vi "SigGen-Compute Max Level (full).vi"(0 "Waveform":T21(xcontrol), 5 "Filter":T4(xcontrol), 9 "Level":T1, 11 "error in (no error)":errorcluster, 12 "Sampling Rate (Hz)":dbl, 13 "Npts":i32) -> (10 "Level out":T1, 14 "Max Level":dbl, 15 "error out":errorcluster)   [LabVIEW 2020]
uses:
  Controls/Waveform XCtl/Waveform XCtl.xctl
  Controls/Advanced Filter XCtl/Advanced Filter XCtl.xctl
  Controls/Level XCtl/Level Data.ctl
  Controls/Level XCtl/Level Units.ctl
  Waveform VIs/Noise VIs/Noise-Globals.vi
  Controls/Level XCtl/Level XCtl.xctl
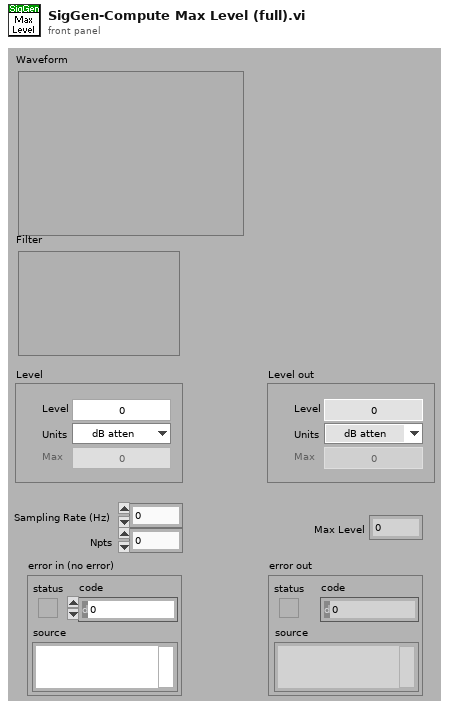
[diagram p1: front panel]
types:
  T1 = typedef "Level XCtl.xctl/Level Data.ctl" = cluster{"Level":dbl, "Units":T2, "Max":dbl, "Multiplier":dbl, "Cal File":path, "Cal":cluster{"Freq (Hz)":dbl[], "Mag (dB SPL)":dbl[], "Phase (deg)":dbl[]}}
  T2 = typedef "Level Units.ctl" = enum16{"dB atten", "dB SPL", "dB re 1 Vrms", "dB V/Hz½", "mW", "dB HL", "Volts", "dB mW"}
  T3 = typedef "Filter-Bandwidth Units.ctl" = enum16{"Linear", "Octaves", "Min-Max"}
  T4 = cluster{"Type":enum16{"Lowpass", "Highpass", "Bandpass", "Bandstop", "OFF"}, "CF (kHz)":dbl, "BW (kHz)":dbl, "Cascade":bool, "Quadrature":bool, "Scale Factor":dbl, "Stages":cluster{"IIR Filter":cluster{"filter structure":enum32{"IIR 2nd Order", "IIR 4th Order"}, "Reverse Coefficients":dbl[], "Forward Coefficients":dbl[]}, "State":dbl[]}[], "Class":enum16{"Elliptic", "Butterworth"}, "Order":i32, "BWUnits":T3}
  T5 = typedef "Waveform Enum.ctl" = enum16{"OFF", "Tone", "Noise", "Pulse Train", "File", "FM Sweep", "Chirp Train", "Complex Tone", "FM Tone", "Moving Ripple"}
  T6 = typedef "Tone Params.ctl" = cluster{"Frequency (kHz)":dbl, "Last Freq":dbl, "Last Phase":dbl}
  T7 = typedef "Pulse Train Params.ctl" = cluster{"Pulse width (us)":dbl, "Pulse rate (Hz)":dbl, "Gap (ms)":dbl, "Polarity":T8, "PT State":T9, "Asynch":bool}
  T8 = typedef "Pulse Polarity.ctl" = enum16{"POS", "NEG", "POS-NEG", "NEG-POS"}
  T9 = typedef "PT-Continuous State.ctl" = cluster{"Template":dbl[], "Nperiod":i32, "Index":i32, "Pulse Rate (Hz)":dbl, "Phase (cycles)":dbl, "Noff":i32}
  T10 = typedef "Noise Params.ctl" = cluster{"InvFilt":bool, "Noise":dbl[], "CurPt":i32, "Aweight":bool, "Seed":i32, "afile":path}
  T11 = typedef "StimFile-Params.ctl" = cluster{"Filename":path, "Signal":dbl[], "Channel":i32, "stream":bool, "offset":i32, "nreps":i32, "loops":i32, "Randomize":bool, "order":i32[], "Seed":i32, "Tokens":i32}
  T12 = typedef "FM Sweep Params.ctl" = cluster{"Rate (oct/s)":dbl, "Fmin (Hz)":dbl, "Fmax (Hz)":dbl, "Ramp (ms)":dbl, "Linear":bool}
  T13 = typedef "Chirp Train.ctl" = cluster{"Params":T14, "Data":cluster{"WF":dbl[]}}
  T14 = typedef "Chirp Train Params.ctl" = cluster{"Fmin (kHz)":dbl, "Fmax (kHz)":dbl, "Compensate":bool, "Duration (ms)":dbl}
  T15 = typedef "CT-Params.ctl" = cluster{"F0 (Hz)":dbl, "Band":cluster{"Flow (Hz)":dbl, "Fhigh (Hz)":dbl}, "Phase":T16, "Min F0 (Hz)":dbl, "Max F0 (Hz)":dbl, "ContinRandPhase":bool, "Max peak factor":dbl, "Max mod depth":dbl, "MinHarmNum":i32, "MaxHarmNum":i32, "Level Mode":enum16{"per component", "overall rms"}, "% jitter":dbl}
  T16 = typedef "CT-Phase Enum.ctl" = enum16{"Cosine", "Random", "Alternating"}
  T17 = typedef "CT-Runtime Data.ctl" = cluster{"Ncomp":i32, "MinHarm":i32, "Phase":dbl[], "Amplitude":dbl[], "Npts/frame":i32, "Last F0":dbl, "Fmin":dbl, "Fmax":dbl, "Lslope":dbl, "randphase":bool, "overall rms":bool, "fmult":dbl[], "jittered":bool}
  T18 = typedef "Moving Ripple.ctl" = cluster{"Params":T19, "Data":T20}
  T19 = typedef "Moving Ripple.Params.ctl" = cluster{"Fmin":dbl, "Fmax":dbl, "Density":dbl, "Velocity":dbl, "Depth":dbl, "Phase":dbl, "Comp/oct":i32}
  T20 = typedef "Moving Ripple.Data.ctl" = cluster{"Freq":dbl[], "A":dbl[], "phase":dbl[], "Phase":dbl}
  T21 = cluster{"Type":T5, "Tone":T6, "Pulse Train":T7, "Noise":T10, "File":T11, "FMSweep":T12, "Chirp Train":T13, "Complex Tone":cluster{"Params":T15, "Data":T17}, "Moving Ripple":T18}
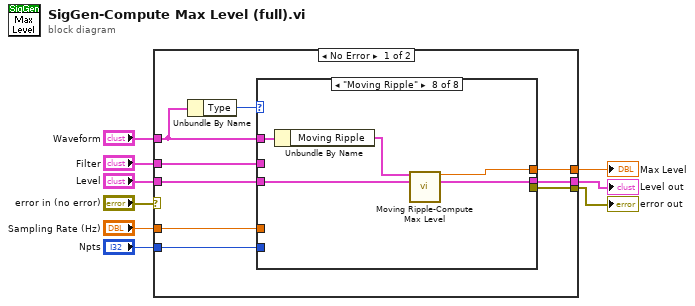
[diagram p0: block diagram]
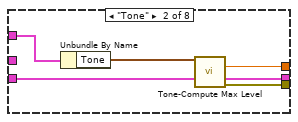
[diagram p3: hidden frame]
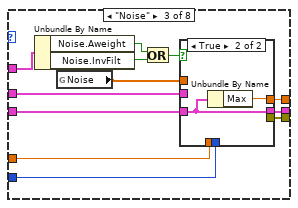
[diagram p4: hidden frame]
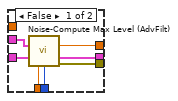
[diagram p5: hidden frame]
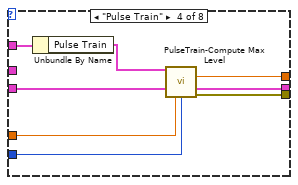
[diagram p6: hidden frame]
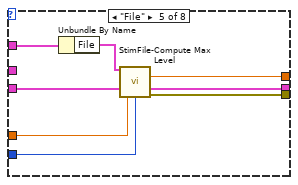
[diagram p7: hidden frame]
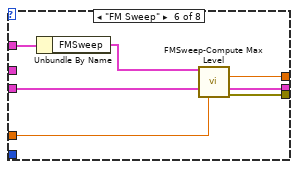
[diagram p8: hidden frame]
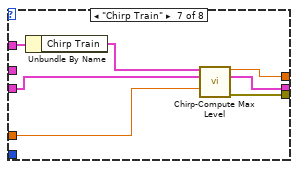
[diagram p9: hidden frame]
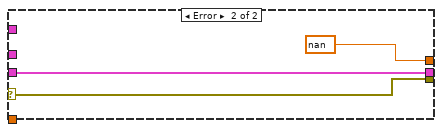
[diagram p10: hidden frame]
diagram:
  n1 = case shown="No Error" "error in (no error)" {
    selector: "error in (no error)" -> [_ w84]
    tunnel: "Level" -> [w16 w82]
    tunnel: "Waveform" -> [w17 _]
    tunnel: "Filter" -> [w13 _]
    tunnel: [w11 w84] -> w8
    tunnel: "Npts" -> [w14 _]
    tunnel: [w10 nan ("Reference Level")] -> w3
    tunnel: "Sampling Rate (Hz)" -> [w15 _]
    tunnel: [w12 w82] -> w1
    frame No Error {
      n2 = Unbundle By Name(w17) -> ("Type"=w18:T5)
      n3 = case shown="\"Moving Ripple\"" w18 {
        tunnel: w17 -> [_ w25 w30 w54 w62 w69 w76 w79]
        tunnel: w16 -> [w19 w23 w37 w49 w57 w65 w70 w81]
        tunnel: w15 -> [_ _ w36 w48 w56 w63 w71 _]
        tunnel: w14 -> [_ _ w35 w47 w55 _ _ _]
        tunnel: w13 -> [_ _ w31 _ _ _ _ _]
        tunnel: [w19 w21 w33 w51 w60 w66 w73 w80] -> w12
        tunnel: [_ w22 w32 w50 w61 w68 w75 _] -> w11
        tunnel: [_ w20 w34 w52 w59 w67 w74 w77] -> w10
        frame "OFF", Default {
        }
        frame "Tone" {
          n4 = Unbundle By Name(w25) -> ("Tone"=w24:T6)
          n5 = call "Tone-Compute Max Level.vi"("Tone Params"=w24, "Level"=w23) -> ("Max Level"=w20:dbl, "Level out"=w21:T1, "error out"=w22:errorcluster)  [unwired: 11 in]
        }
        frame "Noise" {
          n6 = Unbundle By Name(w30) -> ("Noise.Aweight"=w26:bool, "Noise.InvFilt"=w29:bool)
          n7 = global read "Noise-Globals.vi" "Noise"() -> (w28:dbl[])
          n8 = Or(x=w26, y=w29) -> (x .or. y?=w27:bool)
          n9 = case shown="True" w27 {
            tunnel: w37 -> [w44 w46]
            tunnel: w36 -> [w43 _]
            tunnel: w35 -> [w42 _]
            tunnel: [w41 w45] -> w34
            tunnel: [w40 w46] -> w33
            tunnel: [w39 _] -> w32
            tunnel: w31 -> [w38 _]
            tunnel: w28 -> [_ _]
            frame False {
              n10 = call "Noise-Compute Max Level (AdvFilt).vi"("Filter XCtl"=w38, "Level"=w44, "Sampling Rate (Hz)"=w43, "Npts"=w42) -> ("Max Level"=w41:dbl, "Level out"=w40:T1, "error out"=w39:errorcluster)  [unwired: 9 in]
            }
            frame True {
              n11 = Unbundle By Name(w46) -> ("Max"=w45:dbl)
            }
          }
        }
        frame "Pulse Train" {
          n12 = Unbundle By Name(w54) -> ("Pulse Train"=w53:T7)
          n13 = call "PulseTrain-Compute Max Level.vi"("Pulse Train Params"=w53, "Level"=w49, "Sampling Rate (Hz)"=w48, "Npts"=w47) -> ("Max Level"=w52:dbl, "Level out"=w51:T1, "error out"=w50:errorcluster)  [unwired: 9 in]
        }
        frame "File" {
          n14 = Unbundle By Name(w62) -> ("File"=w58:T11)
          n15 = call "StimFile-Compute Max Level.vi"("File"=w58, "Level"=w57, "Sampling Rate (Hz)"=w56, "Npts"=w55) -> ("Max Level"=w59:dbl, "Level out"=w60:T1, "error out"=w61:errorcluster)  [unwired: 9 in]
        }
        frame "FM Sweep" {
          n16 = Unbundle By Name(w69) -> ("FMSweep"=w64:T12)
          n17 = call "FMSweep-Compute Max Level.vi"("FMSweep"=w64, "Level"=w65, "Fs (Hz)"=w63) -> ("Max Level"=w67:dbl, "Level out"=w66:T1, "error out"=w68:errorcluster)  [unwired: 10 in]
        }
        frame "Chirp Train" {
          n18 = Unbundle By Name(w76) -> ("Chirp Train"=w72:T13)
          n19 = call "Chirp-Compute Max Level.vi"("Chirp Train"=w72, "Level in"=w70, "Sampling Rate (Hz)"=w71) -> ("Numeric"=w74:dbl, "Level out"=w73:T1, "error out"=w75:errorcluster)  [unwired: 10 in]
        }
        frame "Moving Ripple" {
          n20 = Unbundle By Name(w79) -> ("Moving Ripple"=w78:T18)
          n21 = call "Moving Ripple-Compute Max Level.vi"("Moving Ripple"=w78, "Level in"=w81) -> ("Max level"=w77:dbl, "Level out"=w80:T1)  [unwired: 12 in]
        }
      }
    }
    frame Error {
    }
  }
  "error out" <- w8
  "Max Level" <- w3
  "Level out" <- w1
